vi "cut_spectrum.vi"(5 "WL Final":dbl, 7 "WL Initial":dbl, 8 "error in":errorcluster, 10 "RL Spectrum":dbl[](array[numeric]), 11 "WL Values":dbl[](array[numeric])) -> (0 "error out":errorcluster, 1 "delta X":dbl, 2 "RL Spectrum":dbl[](array[numeric]), 3 "WL Values":dbl[](array[numeric]))   [LabVIEW 2021]
doc: "Random Laser Project v2.0\nAndré Romero - 2024\nandretec@ifsc.usp.br"
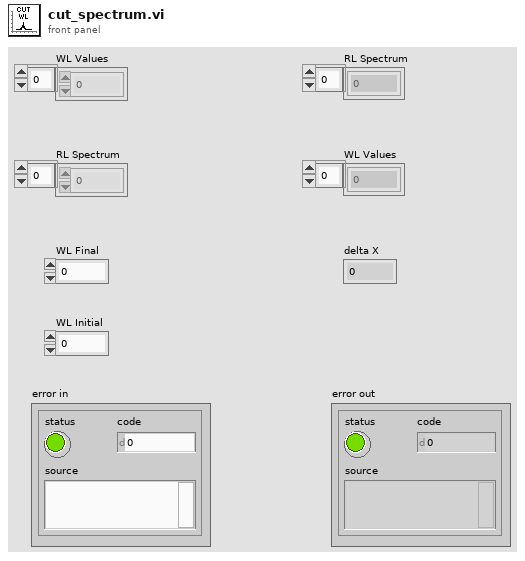
[diagram p1: front panel]
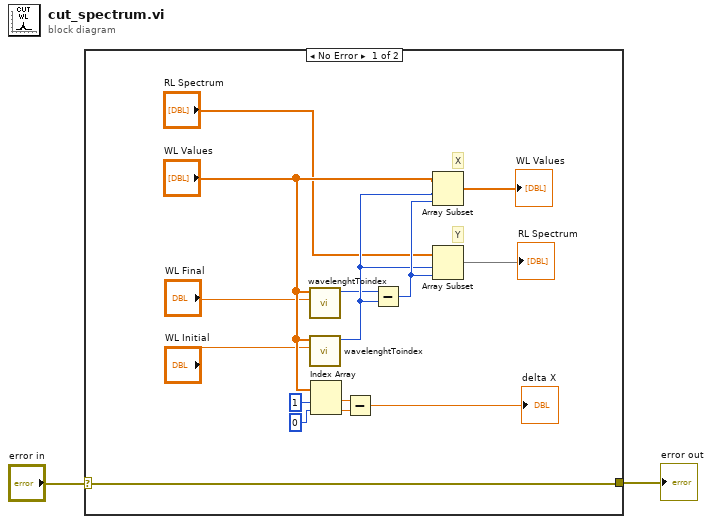
[diagram p0: block diagram]
diagram:
  n1 = case shown="No Error" "error in" {
    selector: "error in" -> [w5 w18]
    tunnel: [w5 w18] -> w1
    frame No Error {
      # "X"
      # "Y"
      n2 = call "wavelenghtToindex.vi"("WL in"="WL Final", "WL Values"="WL Values") -> ("index of WL"=w9:i32)  [unwired: 9 in]
      n3 = call "wavelenghtToindex.vi"("WL in"="WL Initial", "WL Values"="WL Values") -> ("index of WL"=w10:i32)  [unwired: 9 in]
      n4 = Index Array(array="WL Values", index #1=1 ("index"), index #2=0 ("index")) -> (element #1=w15:dbl, element #2=w14:dbl)
      n5 = Subtract(x=w15, y=w14) -> (x-y=→"delta X":dbl)
      n6 = Subtract(x=w9, y=w10) -> (x-y=w11:i32)
      n7 = Array Subset(array="WL Values", index=w10, length=w11) -> (→"WL Values":dbl[])
      n8 = Array Subset(array="RL Spectrum", index=w10, length=w11) -> (→"RL Spectrum":dbl[])
    }
    frame Error {
    }
  }
  "error out" <- w1
